vi "test1.vi"() -> ()   [LabVIEW 2018]
uses:
  <vilib>/express/express analysis/Spectral/Block/exnSpectralBlock spectral measurements peak poly.vi
  <vilib>/express/express analysis/Spectral/Block/exnSpectralBlock spectral measurements peak DDT.vi
  <vilib>/Waveform/WDTOps.llb/WDT Append Waveforms DBL.vi
  <vilib>/Waveform/WDTFileIO.llb/Export Waveform To Spreadsheet File.vi
  <vilib>/express/express analysis/Spectral/XNode/ExpressSpectralMeasurementsBlockNode.xnode
panel:
  in  "stop (F)":bool
  in  "Operating Mode":T1(ring)=enum."Analyze Real-time"
  out "Orignal Signal":dynamicdata(graph)
  in  "Threshold":dbl=0.1
  out "Portion":dynamicdata(graph)
  in  "Portion Duration":i32=200
  out "Index 0":dbl
  out "Index 1":dbl
  out "Index 2":dbl
  out "Index 3":dbl
  out "dt1":dbl
  out "dt2":dbl
  out "dt3":dbl
  in  "Manual depth":dbl=4.3
  in  "Mode":T2(ring)=enum."Use Far Field"
  out "x":dbl format="%#_6f"
  out "y":dbl format="%#_6f"
  out "z":dbl
  in  "peak min":dbl=0.1
  out "ratio":dbl
  out "ratio 2":dbl
  out "ratio 3":dbl
  out "ratio 4":dbl
  out "amplitude":dbl
  out "amplitude 2":dbl
  out "amplitude 3":dbl
  out "amplitude 4":dbl
  out "yaw":dbl
  out "pitch":dbl
  out "Yaw Chart":dbl(graph)
  out "Freq Domain":dynamicdata(graph)
  out "Ratio at Index (%)":dbl
  in  "LPF Cut-Off":dbl=40000.0 caption="Lower Cut-Off"
  out "Selected Index":i32
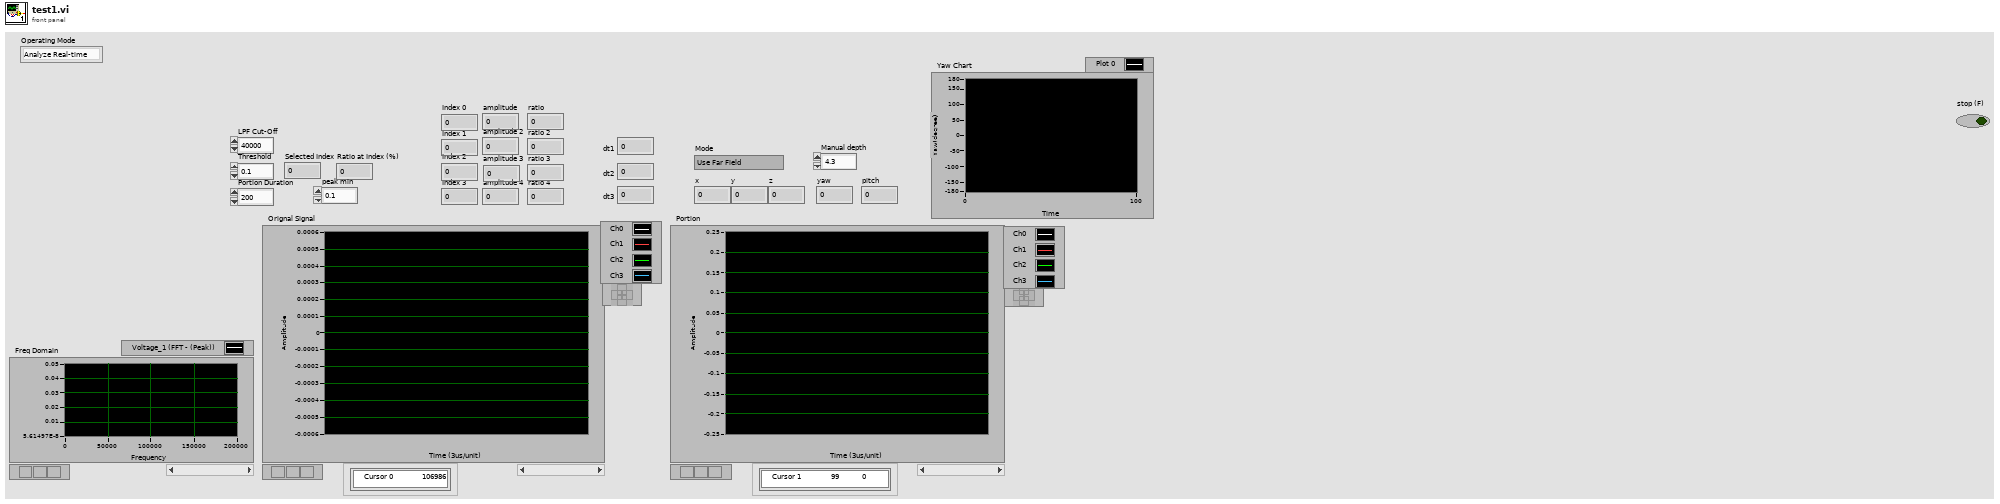
[diagram p1: front panel]
types:
  T1 = enum16{"Analyze From File", "Record Data", "Analyze Real-time"}
  T2 = enum16{"Use Near Field", "Use Far Field", "Send to ROS", "Far Field with 3 hydrophones"}
  T3 = cluster{"averaging mode":u16, "weighting mode":u16, "number of averages":u32}
  T4 = cluster{"dB On (F)":bool, "unwrap phase (F)":bool, "convert to degree (F)":bool}
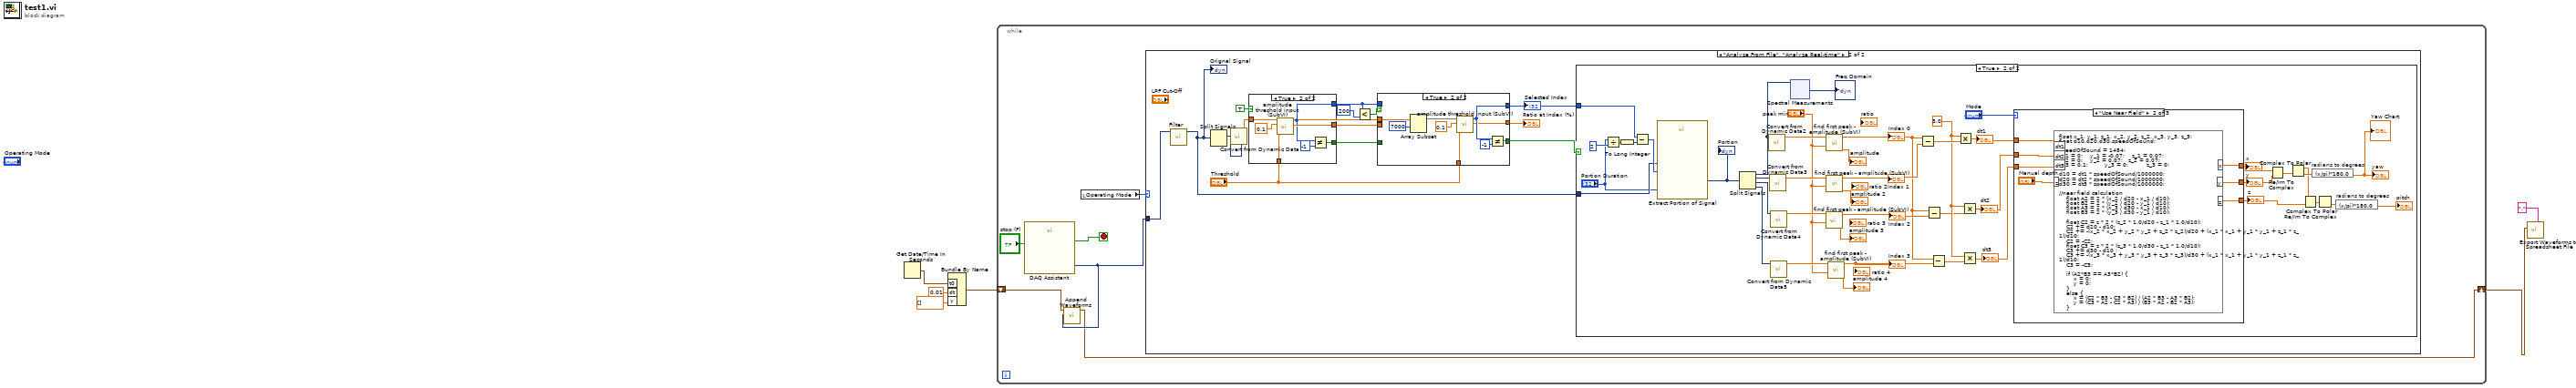
[diagram p0: block diagram]
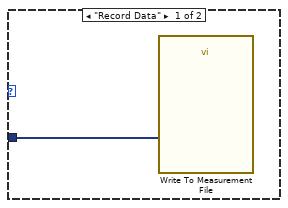
[diagram p2: hidden frame]
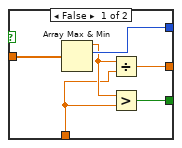
[diagram p4: hidden frame]
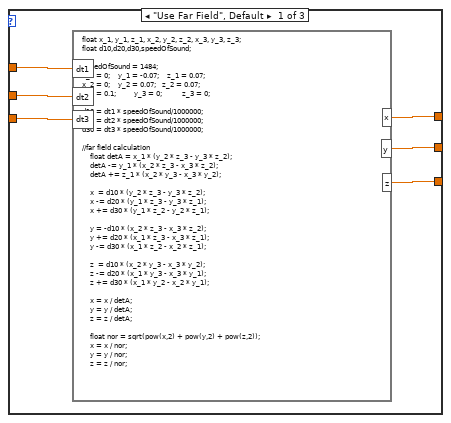
[diagram p6: hidden frame]
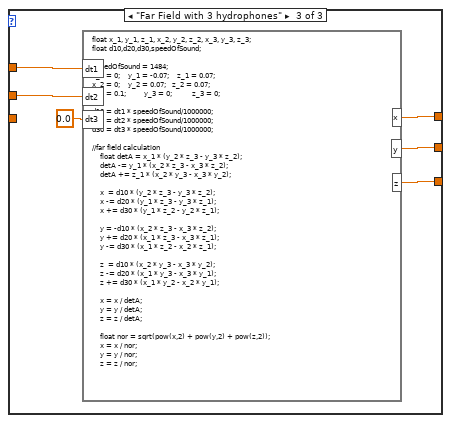
[diagram p7: hidden frame]
diagram:
  n1 = Get Date/Time In Seconds() -> (seconds since 1Jan1904=w6:timestamp)
  n2 = Bundle By Name("t0"=w6, "dt"=0.01, "Y"=dbl[] []) -> (w3:waveform(dbl))  [unwired: 1 in]
  n3 = while {
    shift-right: [w7] -> w1
    shift-left: w3 -> [w9]
    stop <- w11 stop-if-true
    n4 = call "DAQ Assistant"("stop (F)"="stop (F)") -> ("data"=w8:dynamicdata, "stopped"=w11:bool)  [unwired: 15 in, 2 out]
    n5 = call-poly <vilib>:"Append Waveforms.vi"("waveform B"=w8, "waveform A"=w9) -> ("waveform out"=w7:waveform(dbl))  [unwired: 8 in, 1 out]
    n6 = local read "Operating Mode"() -> (w12:T1)
    n7 = case shown="\"Analyze From File\", \"Analyze Real-time\"" w12 {
      tunnel: w8 -> [w13 w16]
      frame "Record Data" {
        n8 = call "Write To Measurement File"("Signals"=w13) -> ()  [unwired: 16 in, 3 out]
      }
      frame "Analyze From File", "Analyze Real-time" {
        n9 = call "Filter"("Signal"=w16) -> ("Filtered Signal"=w15:dynamicdata)  [unwired: 9 in, 1 out]
        "Orignal Signal" <- w15
        n10 = Split Signals(w15) -> (w14:dynamicdata)  [unwired: 4 in, 3 out]
        n11 = call "Convert from Dynamic Data"("Dynamic Data Type"=w14) -> ("Array"=w22:dbl[])  [unwired: 3 in]
        n12 = case shown="True" TRUE {
          tunnel: w22 -> [w45 w52]
          tunnel: [w42 w49] -> w23
          tunnel: [w43 w48] -> w18
          tunnel: [w44 w47] -> w26
          tunnel: "Threshold" -> [w40 w46]
          frame False {
            n13 = Array Max & Min(array=w45) -> (max value=w41:dbl, max index (indices)=w43:i32)  [unwired: 2 out]
            n14 = Divide(x=w41, y=w40) -> (x/y=w42:dbl)
            n15 = Greater?(x=w41, y=w40) -> (0:w44:bool)
          }
          frame True {
            n16 = call "amplitude threshold input (SubVI).vi"("threshold"=w46, "%max amplitude"=0.1, "Array"=w52) -> ("actual ratio (%)"=w49:dbl, "Index"=w48:i32)  [unwired: 7 in]
            n17 = Not Equal?(x=w48, y=-1) -> (x != y?=w47:bool)
          }
        }
        n18 = Less?(x=w18, y=200) -> (x < y?=w24:bool)
        n19 = case shown="True" w24 {
          tunnel: w26 -> [w30 _]
          tunnel: w23 -> [w28 _]
          tunnel: w22 -> [_ w39]
          tunnel: "Threshold" -> [_ w34]
          tunnel: [w30 w33] -> w20
          tunnel: [w29 w32] -> w17
          tunnel: [w28 w31] -> w19
          tunnel: w18 -> [w29 _]
          frame False {
          }
          frame True {
            n20 = Array Subset(array=w39, index=7000) -> (w35:dbl[])  [unwired: 1 in]
            n21 = call "amplitude threshold input (SubVI).vi"("threshold"=w34, "%max amplitude"=0.1, "Array"=w35) -> ("actual ratio (%)"=w31:dbl, "Index"=w32:i32)  [unwired: 7 in]
            n22 = Not Equal?(x=w32, y=-1) -> (x != y?=w33:bool)
          }
        }
        "Ratio at Index (%)" <- w19
        "Selected Index" <- w17
        n23 = case shown="True" w20 {
          tunnel: w15 -> [_ w93]
          tunnel: w17 -> [_ w59]
          frame False {
          }
          frame True {
            w89 = 3.0 ("x")
            n24 = Divide(x="Portion Duration", y=2) -> (x/y=w63:dbl)
            n25 = To Long Integer(number=w63) -> (32bit integer=w62:i32)
            n26 = Subtract(x=w59, y=w62) -> (x-y=w96:i32)
            n27 = call "Extract Portion of Signal"("Samples"="Portion Duration", "Begin Sample"=w96, "Signals"=w93) -> ("Section"=w92:dynamicdata)  [unwired: 7 in, 1 out]
            "Portion" <- w92
            n28 = Split Signals(w92) -> (w53:dynamicdata, w95:dynamicdata, w94:dynamicdata, w91:dynamicdata)  [unwired: 4 in]
            n29 = call "Convert from Dynamic Data2"("Dynamic Data Type"=w53) -> ("Array"=w84:dbl[])  [unwired: 3 in]
            n30 = call "Convert from Dynamic Data3"("Dynamic Data Type"=w95) -> ("Array"=w83:dbl[])  [unwired: 3 in]
            n31 = call "Convert from Dynamic Data4"("Dynamic Data Type"=w94) -> ("Array"=w82:dbl[])  [unwired: 3 in]
            n32 = call "Convert from Dynamic Data5"("Dynamic Data Type"=w91) -> ("Array"=w81:dbl[])  [unwired: 3 in]
            n33 = xnode "Spectral Measurements"("Signals"=w53) -> ("FFT - (Peak)"=→"Freq Domain":dynamicdata)  [unwired: 1 in, 2 out]
            n34 = call "find first peak - amplitude (SubVI).vi"("threshold ratio"="peak min", "Array"=w82) -> ("Peak threshold"=→"amplitude 3":dbl, "Index"=w79:dbl)  [unwired: 5 in, 3 out]
            "Index 2" <- w79
            n35 = call "find first peak - amplitude (SubVI).vi"("threshold ratio"="peak min", "Array"=w84) -> ("Peak threshold"=→"amplitude":dbl, "Index"=w78:dbl)  [unwired: 5 in, 3 out]
            "Index 0" <- w78
            n36 = call "find first peak - amplitude (SubVI).vi"("threshold ratio"="peak min", "Array"=w83) -> ("Peak threshold"=→"amplitude 2":dbl, "Index"=w80:dbl)  [unwired: 5 in, 3 out]
            "Index 1" <- w80
            n37 = call "find first peak - amplitude (SubVI).vi"("threshold ratio"="peak min", "Array"=w81) -> ("Peak threshold"=→"amplitude 4":dbl, "Index"=w77:dbl)  [unwired: 5 in, 3 out]
            "Index 3" <- w77
            n38 = Subtract(x=w78, y=w80) -> (x-y=w90:dbl)
            n39 = Subtract(x=w78, y=w79) -> (x-y=w88:dbl)
            n40 = Subtract(x=w78, y=w77) -> (x-y=w87:dbl)
            n41 = Multiply(x=w89, y=w90) -> (x*y=w66:dbl)
            "dt1" <- w66
            n42 = Multiply(x=w89, y=w88) -> (x*y=w86:dbl)
            "dt2" <- w86
            n43 = Multiply(x=w89, y=w87) -> (x*y=w65:dbl)
            "dt3" <- w65
            n44 = case shown="\"Use Near Field\"" "Mode" {
              tunnel: w66 -> [w112 w119 w125]
              tunnel: w86 -> [w111 w118 w124]
              tunnel: [w110 w117 w122] -> w73
              tunnel: [w109 w116 w121] -> w72
              tunnel: [w108 w115 w120] -> w71
              tunnel: w65 -> [w107 w113 _]
              frame "Use Far Field", Default {
                n45 = formula code="float x_1, y_1, z_1, x_2, y_2, z_2, x_3, y_3, z_3;\nfloat d10,d20,d30,speedOfSound;\n\nspeedOfSound = 1484;\nx_1 = 0;    y_1 = -0.07;    z_1 = 0.07;\nx_2 = 0;    y_2 = 0.07;   z_2 = 0.07;\nx_3 = 0.1;         y_3 = 0;          z_3 = 0;\n\nd10 = dt1 * speedOfSound/1000000;\nd20 = dt2 * speedOfSound/1000000;\nd30 = dt3 * speedOfSound/1000000;\n\n//far field calculation\n    float detA = x_1 * (y_2 * z_3 - y_3 * z_2);\n    detA -= y_1 * (x_2 * z_3 - x_3 * z_2);\n    detA += z_1 * (x_2 * y_3 - x_3 * y_2);\n\n    x  = d10 * (y_2 * z_3 - y_3 * z_2);\n    x -= d20 * (y_1 * z_3 - y_3 * z_1);\n    x += d30 * (y_1 * z_2 - y_2 * z_1);\n\n    y = -d10 * (x_2 * z_3 - x_3 * z_2);\n    y += d20 * (x_1 * z_3 - x_3 * z_1);\n    y -= d30 * (x_1 * z_2 - x_2 * z_1);\n\n    z  = d10 * (x_2 * y_3 - x_3 * y_2);\n    z -= d20 * (x_1 * y_3 - x_3 * y_1);\n    z += d30 * (x_1 * y_2 - x_2 * y_1);\n\n    x = x / detA;\n    y = y / detA;\n    z = z / detA;\n\n    float nor = sqrt(pow(x,2) + pow(y,2) + pow(z,2));\n    x = x / nor;\n    y = y / nor;\n    z = z / nor;"("dt1"=w112, "dt2"=w111, "dt3"=w107) -> ("x"=w110:dbl, "y"=w109:dbl, "z"=w108:dbl)
              }
              frame "Use Near Field" {
                n46 = formula code="float x_1, y_1, z_1, x_2, y_2, z_2, x_3, y_3, z_3;\nfloat d10,d20,d30,speedOfSound;\n\nspeedOfSound = 1484;\nx_1 = 0;    y_1 = -0.07;    z_1 = 0.07;\nx_2 = 0;    y_2 = 0.07;   z_2 = 0.07;\nx_3 = 0.1;         y_3 = 0;          z_3 = 0;\n\nd10 = dt1 * speedOfSound/1000000;\nd20 = dt2 * speedOfSound/1000000;\nd30 = dt3 * speedOfSound/1000000;\n\n//near field calculation\n    float A2 = 2 * (x_2 / d20 - x_1 / d10);\n    float B2 = 2 * (y_2 / d20 - y_1 / d10);\n    float A3 = 2 * (x_3 / d30 - x_1 / d10);\n    float B3 = 2 * (y_3 / d30 - y_1 / d10);\n    \n    float C2 = z * 2 * (z_2 * 1.0/d20 - z_1 * 1.0/d10);\n    C2 += d20 - d10;\n    C2 += -(x_2 * x_2 + y_2 * y_2 + z_2 * z_2)/d20 + (x_1 * x_1 + y_1 * y_1 + z_1 * z_1)/d10;\n    C2 = -C2;\n    float C3 = z * 2 * (z_3 * 1.0/d30 - z_1 * 1.0/d10);\n    C3 += d30 - d10 ;\n    C3 += -(x_3 * x_3 + y_3 * y_3 + z_3 * z_3)/d30 + (x_1 * x_1 + y_1 * y_1 + z_1 * z_1)/d10;\n    C3 = -C3;\n\n    if (A2*B3 == A3*B2) {\n        x = 0;\n        y = 0;\n    }\n    else {\n        x = (C2 * B3 - C3 * B2) / (A2 * B3 - A3 * B2);\n        y = (C3 * A2 - C2 * A3) / (B3 * A2 - B2 * A3);\n    }"("dt1"=w119, "dt2"=w118, "dt3"=w113, "z"="Manual depth") -> ("x"=w117:dbl, "y"=w116:dbl, "z"=w115:dbl)
              }
              frame "Far Field with 3 hydrophones" {
                n47 = formula code="float x_1, y_1, z_1, x_2, y_2, z_2, x_3, y_3, z_3;\nfloat d10,d20,d30,speedOfSound;\n\nspeedOfSound = 1484;\nx_1 = 0;    y_1 = -0.07;    z_1 = 0.07;\nx_2 = 0;    y_2 = 0.07;   z_2 = 0.07;\nx_3 = 0.1;         y_3 = 0;          z_3 = 0;\n\nd10 = dt1 * speedOfSound/1000000;\nd20 = dt2 * speedOfSound/1000000;\nd30 = dt3 * speedOfSound/1000000;\n\n//far field calculation\n    float detA = x_1 * (y_2 * z_3 - y_3 * z_2);\n    detA -= y_1 * (x_2 * z_3 - x_3 * z_2);\n    detA += z_1 * (x_2 * y_3 - x_3 * y_2);\n\n    x  = d10 * (y_2 * z_3 - y_3 * z_2);\n    x -= d20 * (y_1 * z_3 - y_3 * z_1);\n    x += d30 * (y_1 * z_2 - y_2 * z_1);\n\n    y = -d10 * (x_2 * z_3 - x_3 * z_2);\n    y += d20 * (x_1 * z_3 - x_3 * z_1);\n    y -= d30 * (x_1 * z_2 - x_2 * z_1);\n\n    z  = d10 * (x_2 * y_3 - x_3 * y_2);\n    z -= d20 * (x_1 * y_3 - x_3 * y_1);\n    z += d30 * (x_1 * y_2 - x_2 * y_1);\n\n    x = x / detA;\n    y = y / detA;\n    z = z / detA;\n\n    float nor = sqrt(pow(x,2) + pow(y,2) + pow(z,2));\n    x = x / nor;\n    y = y / nor;\n    z = z / nor;"("dt1"=w125, "dt2"=w124, "dt3"=0.0 ("input variable")) -> ("x"=w122:dbl, "y"=w121:dbl, "z"=w120:dbl)
              }
            }
            "x" <- w73
            "y" <- w72
            "z" <- w71
            n48 = Re/Im To Complex(1:w72, 2:w73) -> (0:w75:cdb)
            n49 = Complex To Polar(r * e^(i*theta)=w75) -> (r=w70:dbl, theta=w74:dbl)
            n50 = Re/Im To Complex(1:w71, 2:w70) -> (0:w69:cdb)
            n51 = expression code="(x/pi)*180.0" "radians to degrees"(w74) -> (→"yaw" →"Yaw Chart":dbl)
            n52 = Complex To Polar(r * e^(i*theta)=w69) -> (theta=w67:dbl)  [unwired: 1 out]
            n53 = expression code="(x/pi)*180.0" "radians to degrees"(w67) -> (→"pitch":dbl)
          }
        }
      }
    }
  }
  n54 = call-poly <vilib>:"Export Waveforms to Spreadsheet File.vi"("delimiter (Tab)"=".", "waveform"=w1) -> ()  [unwired: 8 in, 2 out]
